vi "sv_STFT by Increment (Waterfall).vi"(0 "scaled signal [EU]":waveform(dbl), 1 "weighting filter":T5 items=["Linear", "A-weighting", "B-weighting", "C-weighting", "ITU-R 468-4", "Dolby", "CCITT", "C-message", "Wb", "Wc", "Wd", "We", "Wf", "Wh", "Wj", "Wk", "Wm", "AES17 20 kHz lowpass", "AES17 40 kHz lowpass", "AES17 20 kHz highpass", "AES17 40 kHz highpass"], 7 "FFT info":T7={"FFT block size"=1024, "number of FFT"=0, "start index"=0, "increment"=0.0} {"increment" format="%.2f"}, 11 "error in (no error)":errorcluster, 12 "window":T8(ring)=enum."Hanning", 13 "dB On (T)":bool=TRUE) -> (4 "power spectra":cluster{"x0":dbl, "dx":dbl, "Y":dbl[]}[](array[cluster]), 6 "unit label":string, 10 "spectrum info":T1={"channel name"="", "description"="", "x-axis units"=0, "spectral info"={"spectrum type"=enum."Power [Magnitude^2]", "linear/dB"=enum."linear", "window"=0, "window size"=0, "FFT size"=0}, "engineering units"=0, "custom label"="", "dB reference [EU]"=0.0, "peak units"=enum."rms", "weighting filter"=0, "spectral density?"=FALSE, "unit label"="", "spectrum skewed?"=FALSE, "complimentary spectrum units"=enum."none"} {"x-axis units" items=["Time (s)"=0, "Frequency-CB (Hz)"=1, "Frequency-CPB (Hz)"=1248, "Frequency-Arbitrary (Hz)"=2357, "Quefrency (s)"=2, "Revolutions (rev)"=3, "Order"=4, "Speed (RPM)"=11, "Speed (rad/s)"=21, "Index"=65535]; "weighting filter" items=["Linear", "A-weighting", "B-weighting", "C-weighting", "ITU-R 468-4", "Dolby", "CCITT", "C-message", "Wb", "Wc", "Wd", "We", "Wf", "Wh", "Wj", "Wk", "Wm", "AES17 20 kHz lowpass", "AES17 40 kHz lowpass", "AES17 20 kHz highpass", "AES17 40 kHz highpass"]; "dB reference [EU]" format="%.2f"; "engineering units" items=["custom..."=0, "V"=1, "A"=21, "C"=30, "pC"=31, "s"=32, "-"=29, "Pa"=2, "N"=20, "g"=3, "m/s^2"=4, "m/s"=5, "m"=6, "mm/s"=12, "mm"=13, "micron/s"=14, "micron"=15, "in/s^2"=7, "in/s"=8, "in"=9, "mil/s"=10, "mil"=11, "rad/s^2"=16, "rad/s"=17, "rad"=18, "deg/s^2"=26, "deg/s"=27, "deg"=28, "RPM"=22, "cycle/s^2"=23, "Hz"=24, "cycle"=25, "strain"=19]; "spectral info"."window" items=["None "=0, "Hanning"=1, "Hamming"=2, "Blackman-Harris"=3, "Exact Blackman"=4, "Blackman"=5, "Flat Top"=6, "4 Term B-Harris "=7, "7 Term B-Harris"=8, "Low Sidelobe"=9, "Force - Exponential"=10, "Gaussian"=62]}, 15 "error out":errorcluster)   [LabVIEW 2017, in "SoundVib_Transient.lvlib"]
uses:
  <vilib>/addons/Sound and Vibration/svt_Transients/SoundVib_Transient.lvlib
  <vilib>/addons/_NISVFA/_Shared subVIs/Controls/svc_Weighting Filter Text Ring.ctl
  <vilib>/addons/_NISVFA/_Shared subVIs/Controls/svc_Spectrum Info.ctl
  <vilib>/addons/_NISVFA/_Shared subVIs/Controls/svc_X-Axis Units.ctl
  <vilib>/addons/_NISVFA/_Shared subVIs/Controls/svc_Spectrum Type.ctl
  <vilib>/addons/_NISVFA/_Shared subVIs/Controls/svc_Engineering Units Text Ring.ctl
  <vilib>/addons/_NISVFA/_Shared subVIs/Controls/svc_Complimentary Spectrum Units.ctl
  <vilib>/addons/Sound and Vibration/svt_Weighting/SVT Weighting Filter (frequency) (1 Ch).vi
  <vilib>/addons/_NISVFA/_Baseband FFT/SVFA Power Spectrum (1 Ch).vi
  <vilib>/addons/Sound and Vibration/svt_Weighting/SoundVib_ABCWeighting.lvlib
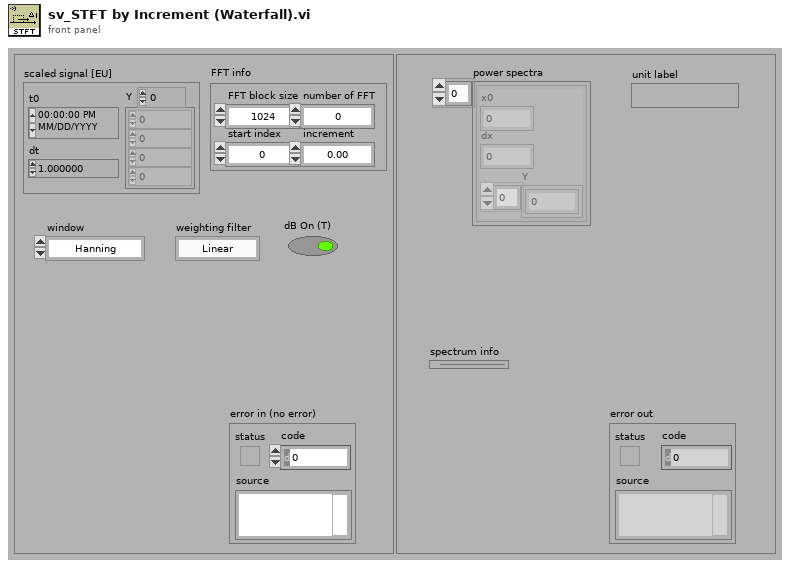
[diagram p1: front panel]
types:
  T1 = typedef "svc_Spectrum Info.ctl" = cluster{"channel name":string, "description":string, "x-axis units":T2, "spectral info":cluster{"spectrum type":T3, "linear/dB":enum16{"linear", "dB"}, "window":u16, "window size":i32, "FFT size":i32}, "engineering units":T4, "custom label":string, "dB reference [EU]":dbl, "peak units":enum16{"rms", "peak", "peak-peak"}, "weighting filter":T5, "spectral density?":bool, "unit label":string, "spectrum skewed?":bool, "complimentary spectrum units":T6}
  T2 = typedef "svc_X-Axis Units.ctl" = u16
  T3 = typedef "svc_Spectrum Type.ctl" = enum16{"FFT Spectrum [complex]", "Amplitude [Magnitude]", "Power [Magnitude^2]", "Cross Spectrum [complex]", "Frequency Response [Complex]"}
  T4 = typedef "svc_Engineering Units Text Ring.ctl" = u16
  T5 = typedef "svc_Weighting Filter Text Ring.ctl" = u16
  T6 = typedef "svc_Complimentary Spectrum Units.ctl" = enum16{"none", "radians", "degrees", "cycles", "imaginary"}
  T7 = cluster{"FFT block size":i32, "number of FFT":i32, "start index":i32, "increment":dbl}
  T8 = enum16{"None ", "Hanning", "Hamming", "Blackman-Harris", "Exact Blackman", "Blackman", "Flat Top", "4 Term B-Harris ", "7 Term B-Harris", "Low Sidelobe"}
  T9 = cluster{"averaging mode":enum16{"No averaging", "Vector averaging", "RMS averaging", "Peak hold"}, "weighting mode":enum16{"Linear", "Exponential"}, "number of averages":u32, "linear mode":enum16{"One shot", "Auto restart"}}
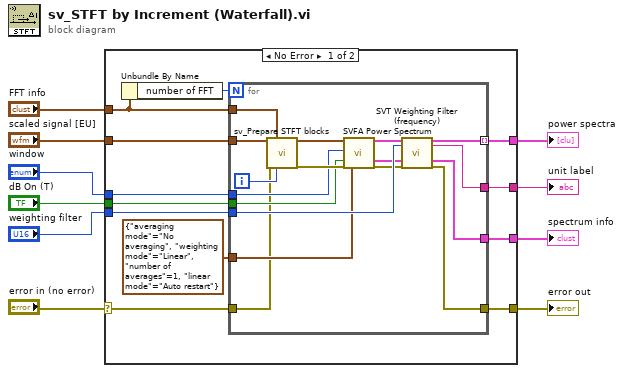
[diagram p0: block diagram]
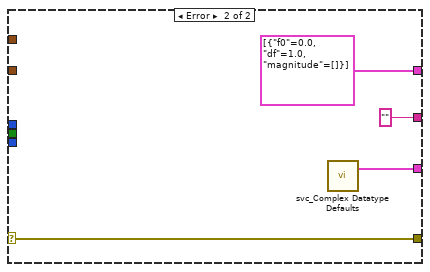
[diagram p2: hidden frame]
diagram:
  n1 = case shown="No Error" "error in (no error)" {
    selector: "error in (no error)" -> [w14 w43]
    tunnel: "dB On (T)" -> [w22 _]
    tunnel: "window" -> [w21 _]
    tunnel: "scaled signal [EU]" -> [w20 _]
    tunnel: "weighting filter" -> [w19 _]
    tunnel: [w18 "" ("unit label")] -> w6
    tunnel: "FFT info" -> [w17 _]
    tunnel: [w13 w43] -> w3
    tunnel: [w12 cluster{"f0":dbl, "df":dbl, "magnitude":dbl[]}[] [{"f0"=0.0, "df"=1.0, "magnitude"=[]}]] -> w2
    tunnel: [w11 w40] -> w1
    frame No Error {
      n2 = Unbundle By Name(w17) -> ("number of FFT"=w16:i32)
      n3 = for {
        N: w16 -> [_]
        tunnel: w22 -> [w29]
        tunnel: w21 -> [w28]
        tunnel: w20 -> [w39]
        tunnel: w17 -> [w38]
        tunnel: w19 -> [w36]
        tunnel: [w24] -> w12 mode=indexing
        tunnel: [w35] -> w18
        tunnel: T9 {"averaging mode"=enum."No averaging", "weighting mode"=enum."Linear", "number of averages"=1, "linear mode"=enum."Auto restart"} ("averaging parameters") -> [w27]
        tunnel: w14 -> [w26]
        tunnel: [w25] -> w13
        tunnel: [w23] -> w11
        i -> [w37]
        n4 = call <vilib>:"sv_Prepare STFT blocks.vi"("scaled signal [EU]"=w39, "FFT info"=w38, "error in (no error)"=w26, "iteration"=w37) -> ("scaled signal [EU]"=w34:waveform(dbl), "error out"=w30:errorcluster)  [unwired: 10 in]
        n5 = call-poly <vilib>:"SVFA Power Spectrum.vi"("scaled signal [EU]"=w34, "window"=w28, "dB On (T)"=w29, "error in (no error)"=w30, "averaging parameters"=w27) -> ("power spectrum [dB EU]"=w33:cluster{"f0":dbl, "df":dbl, "magnitude":dbl[]}, "spectrum info"=w31:T1, "error out"=w32:errorcluster)  [unwired: 9 in, 3 out]
        n6 = call-poly <vilib>:"SVT Weighting Filter (frequency).vi"("spectrum"=w33, "weighting"=w36, "spectrum info in"=w31, "error in (no error)"=w32) -> ("weighted spectrum"=w24:cluster{"f0":dbl, "df":dbl, "magnitude":dbl[]}, "unit label"=w35:string, "spectrum info out"=w23:T1, "error out"=w25:errorcluster)  [unwired: 12 in]
      }
    }
    frame Error {
      n7 = call <vilib>:"svc_Complex Datatype Defaults.vi"() -> ("dead spectrum info"=w40:T1)  [unwired: 11 in, 8 out]
    }
  }
  "unit label" <- w6
  "error out" <- w3
  "power spectra" <- w2
  "spectrum info" <- w1
